vi "flatten.vi"(8 "error in":errorcluster, 11 "test-system in":refnum<class "test-system.lvclass">) -> (0 "error out":errorcluster, 2 "flattened system":string, 3 "test-system out":refnum<class "test-system.lvclass">)   [LabVIEW 2020, in "test-system.lvclass"]
uses:
  test-system.lvclass
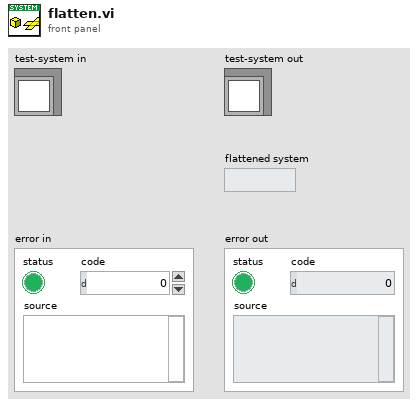
[diagram p1: front panel]
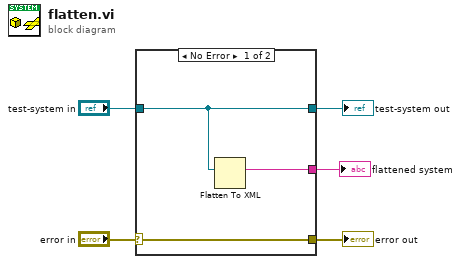
[diagram p0: block diagram]
diagram:
  n1 = case shown="No Error" "error in" {
    selector: "error in" -> [w8 w10]
    tunnel: [w8 w10] -> w4
    tunnel: [w7 w9] -> w2
    tunnel: "test-system in" -> [w7 w9]
    tunnel: [w6 _] -> w1
    frame No Error {
      n2 = Flatten To XML(6:w7) -> (2:w6:string)
    }
    frame Error {
    }
  }
  "error out" <- w4
  "test-system out" <- w2
  "flattened system" <- w1
